vi "Check Value Type.vi"(8 "error in (no error)":errorcluster, 11 "Timestamp Column in":refnum<class "Timestamp Column.lvclass">) -> (0 "error out":errorcluster, 3 "Timestamp Column out":refnum<class "Timestamp Column.lvclass">)   [LabVIEW 2020, in "Basic Columns.lvlib" / "Timestamp Column.lvclass"]
uses:
  Timestamp Column.lvclass
  Timestamp Column.lvclass/Timestamp Column.ctl
  Column Interface/Timestamp Rule Interface/Timestamp Rule Interface.lvclass
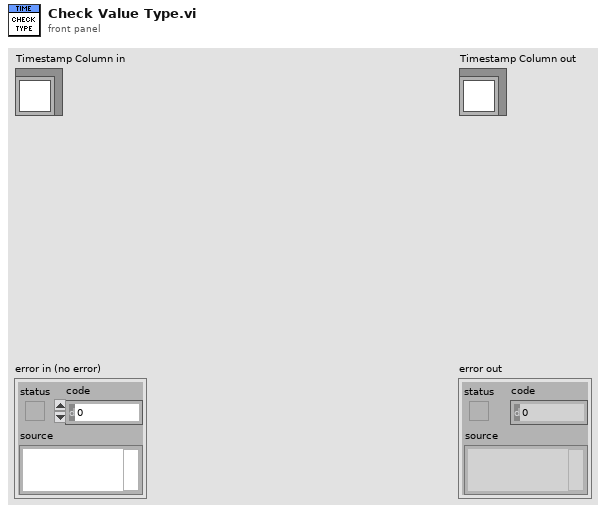
[diagram p1: front panel]
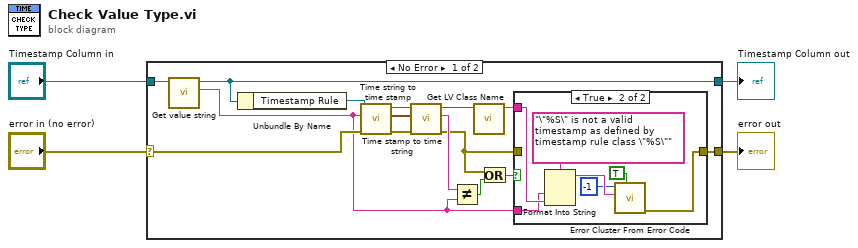
[diagram p0: block diagram]
diagram:
  n1 = case shown="No Error" "error in (no error)" {
    selector: "error in (no error)" -> [w10 w28]
    tunnel: "Timestamp Column in" -> [w19 w29]
    tunnel: [w18 w29] -> w2
    tunnel: [w5 w28] -> w1
    frame No Error {
      n2 = call-dynamic "Get value string.vi"("Column in"=w19) -> ("Value"=w7:string, "Column out"=w18:refnum<class "Timestamp Column.lvclass">)  [unwired: 8 in, 1 out]
      n3 = Unbundle By Name(w18) -> ("Timestamp Rule"=w17:refnum<class "Timestamp Rule Interface.lvclass">)
      n4 = call-dynamic "Time string to time stamp.vi"("error in (no error)"=w10, "Time String"=w7, "Timestamp Rule Interface in"=w17) -> ("error out"=w12:errorcluster, "Time Stamp"=w16:timestamp, "Timestamp Rule Interface out"=w15:refnum<class "Timestamp Rule Interface.lvclass">)  [unwired: 6 in]
      n5 = call-dynamic "Time stamp to time string.vi"("error in (no error)"=w12, "Time Stamp"=w16, "Timestamp Rule Interface in"=w15) -> ("error out"=w6:errorcluster, "String"=w14:string, "Timestamp Rule Interface out"=w9:refnum<class "Timestamp Rule Interface.lvclass">)  [unwired: 6 in]
      n6 = Not Equal?(x=w14, y=w7) -> (x != y?=w13:bool)
      n7 = call <vilib>:"Get LV Class Name.vi"("object"=w9) -> ("class name"=w8:string)  [unwired: 9 in, 1 out]
      n8 = Or(x=w6, y=w13) -> (x .or. y?=w11:bool)
      n9 = case shown="True" w11 {
        tunnel: w8 -> [_ w26]
        tunnel: w7 -> [_ w25]
        tunnel: w6 -> [w20 _]
        tunnel: [w20 w21] -> w5
        frame False {
        }
        frame True {
          n10 = Format Into String(format string="\"%S\" is not a valid timestamp as defined by timestamp rule class \"%S\"", w25, w26) -> (resulting string=w24:string)  [unwired: 2 in, 1 out]
          n11 = call <vilib>:"Error Cluster From Error Code.vi"("show call chain? (False)"=TRUE, "error message (\"\")"=w24, "error code (0)"=-1) -> ("error out"=w21:errorcluster)  [unwired: 6 in]
        }
      }
    }
    frame Error {
    }
  }
  "error out" <- w1
  "Timestamp Column out" <- w2
